vi "Feeder_teleop.vi"(11 "Joystick Controls":T1) -> ()   [LabVIEW 2020]
uses:
  Utility VIs/Joystick_Controls.ctl
  Systems/Feeder/Feeder_Cluster.ctl
  Systems/Feeder/Feeder_Control_States.ctl
  Globals/Feeder_Globals.vi
panel:
  in  "funnel_throttle":dbl=0.6
  in  "Magazine_Power":dbl=0.5
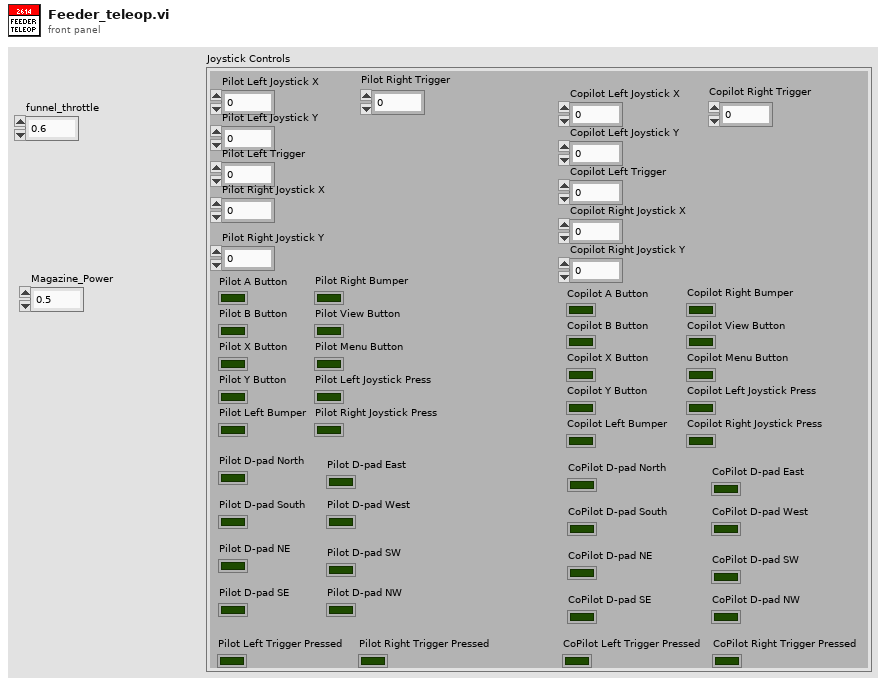
[diagram p1: front panel]
types:
  T1 = typedef "Joystick_Controls.ctl" = cluster{"Pilot Left Joystick X":dbl, "Pilot Left Joystick Y":dbl, "Pilot A Button":bool, "Pilot B Button":bool, "Pilot X Button":bool, "Pilot Y Button":bool, "Pilot Left Bumper":bool, "Pilot Right Bumper":bool, "Pilot View Button":bool, "Pilot Menu Button":bool, "Pilot Left Joystick Press":bool, "Pilot Right Joystick Press":bool, "Pilot Left Trigger":dbl, "Pilot Right Joystick X":dbl, "Pilot Right Joystick Y":dbl, "Pilot Right Trigger":dbl, "Copilot Left Joystick X":dbl, "Copilot Left Joystick Y":dbl, "Copilot A Button":bool, "Copilot B Button":bool, "Copilot X Button":bool, "Copilot Y Button":bool, "Copilot Left Bumper":bool, "Copilot Right Bumper":bool, "Copilot View Button":bool, "Copilot Menu Button":bool, "Copilot Left Joystick Press":bool, "Copilot Right Joystick Press":bool, "Copilot Left Trigger":dbl, "Copilot Right Joystick X":dbl, "Copilot Right Joystick Y":dbl, "Copilot Right Trigger":dbl, "Pilot D-pad North":bool, "Pilot D-pad South":bool, "Pilot D-pad East":bool, "Pilot D-pad West":bool, "Pilot D-pad NE ":bool, "Pilot D-pad SE":bool, "Pilot D-pad SW":bool, "Pilot D-pad NW":bool, "CoPilot D-pad North":bool, "CoPilot D-pad South":bool, "CoPilot D-pad East":bool, "CoPilot D-pad West":bool, "CoPilot D-pad NE":bool, "CoPilot D-pad SE":bool, "CoPilot D-pad SW":bool, "CoPilot D-pad NW":bool, "Pilot Left Trigger Pressed":bool, "Pilot Right Trigger Pressed":bool, "CoPilot Left Trigger Pressed":bool, "CoPilot Right Trigger Pressed":bool}
  T2 = typedef "Feeder_Cluster.ctl" = cluster{"Firing":bool, "Load":bool, "Magazine_%Vbus":dbl, "Funnel_%Vbus":dbl, "Intake_%Vbus":dbl, "Manual_Extend":bool, "Outtake":bool, "Parameters":dbl[], "Auto_Notifier":refnum<notifier>, "Step":i32, "Control_States":T3}
  T3 = typedef "Feeder_Control_States.ctl" = enum16{"No-Op", "Manual", "Load", "Outtake", "Firing", "Test"}
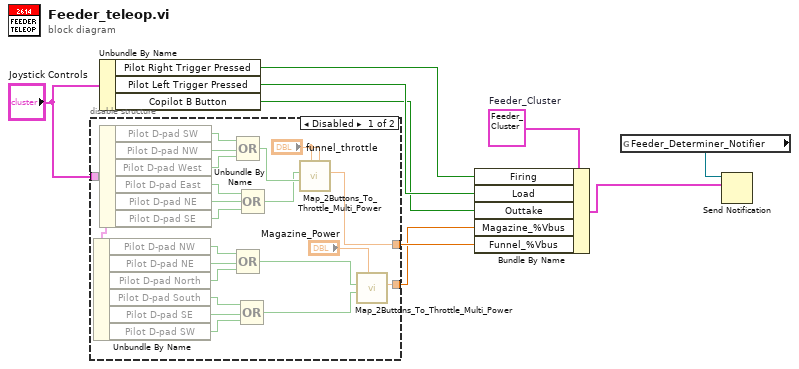
[diagram p0: block diagram]
diagram:
  w2 = T2 {"Firing"=FALSE, "Load"=FALSE, "Magazine_%Vbus"=0.0, "Funnel_%Vbus"=0.0, "Intake_%Vbus"=0.0, "Manual_Extend"=FALSE, "Outtake"=FALSE, "Parameters"=[], "Auto_Notifier"=refnum, "Step"=0, "Control_States"=enum."No-Op"}  # Feeder_Cluster
  n1 = disable-structure shown="Disabled" {
    disable-tunnel: "Joystick Controls" -> [w22 _]
    disable-tunnel: [w30 _] -> w9
    disable-tunnel: [w14 _] -> w8
    frame Disabled {
      n2 = Unbundle By Name(w22) -> ("Pilot D-pad NW"=w21:bool, "Pilot D-pad NE"=w20:bool, "Pilot D-pad North"=w19:bool, "Pilot D-pad South"=w18:bool, "Pilot D-pad SE"=w17:bool, "Pilot D-pad SW"=w16:bool)
      n3 = Unbundle By Name(w22) -> ("Pilot D-pad SW"=w28:bool, "Pilot D-pad NW"=w27:bool, "Pilot D-pad West"=w26:bool, "Pilot D-pad East"=w25:bool, "Pilot D-pad NE"=w24:bool, "Pilot D-pad SE"=w23:bool)
      n4 = Compound Arithmetic op=OR(w28, w27, w26) -> (w29:bool)
      n5 = Compound Arithmetic op=OR(w21, w20, w19) -> (w13:bool)
      n6 = Compound Arithmetic op=OR(w18, w17, w16) -> (w15:bool)
      n7 = Compound Arithmetic op=OR(w25, w24, w23) -> (w11:bool)
      n8 = call "Map_2Buttons_To_Throttle_Multi_Power.vi"("Power_Down"="funnel_throttle", "Power_Up"="funnel_throttle", "Down"=w29, "Up"=w11) -> ("Throttle"=w30:dbl)  [unwired: 7 in]
      n9 = call "Map_2Buttons_To_Throttle_Multi_Power.vi"("Power_Up"="Magazine_Power", "Down"=w15, "Up"=w13) -> ("Throttle"=w14:dbl)  [unwired: 8 in]
    }
    frame Enabled {
    }
  }
  n10 = Unbundle By Name("Joystick Controls") -> ("Pilot Right Trigger Pressed"=w5:bool, "Pilot Left Trigger Pressed"=w4:bool, "Copilot B Button"=w3:bool)
  n11 = Bundle By Name(cluster=w2, "Firing"=w5, "Load"=w4, "Outtake"=w3, "Magazine_%Vbus"=w8, "Funnel_%Vbus"=w9) -> (w6:T2)
  n12 = global read "Feeder_Globals.vi" "Feeder_Determiner_Notifier"() -> (w1:refnum<notifier>)
  n13 = Send Notification(notification=w6, notifier=w1) -> ()  [unwired: 1 in, 2 out]
